vi "Eurotherm_read_TH.vi"(0 "Modbus Master in":refnum<class "Modbus Master.lvclass">, 5 "error in (no error)":errorcluster) -> (12 "HR_rd":dbl min=-28.0 max=70.0 step=0.1, 14 "Modbus Master out":refnum<class "Modbus Master.lvclass">, 18 "Tª_rd":dbl min=-28.0 max=70.0 step=0.1, 19 "error out":errorcluster)   [LabVIEW 2021, in "CC_Library.lvlib"]
uses:
  CC_Library.lvlib
  <vilib>/Modbus/master/Modbus Master.lvclass
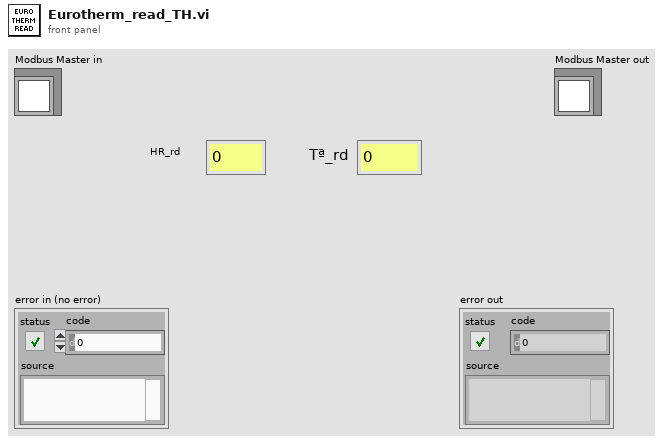
[diagram p1: front panel]
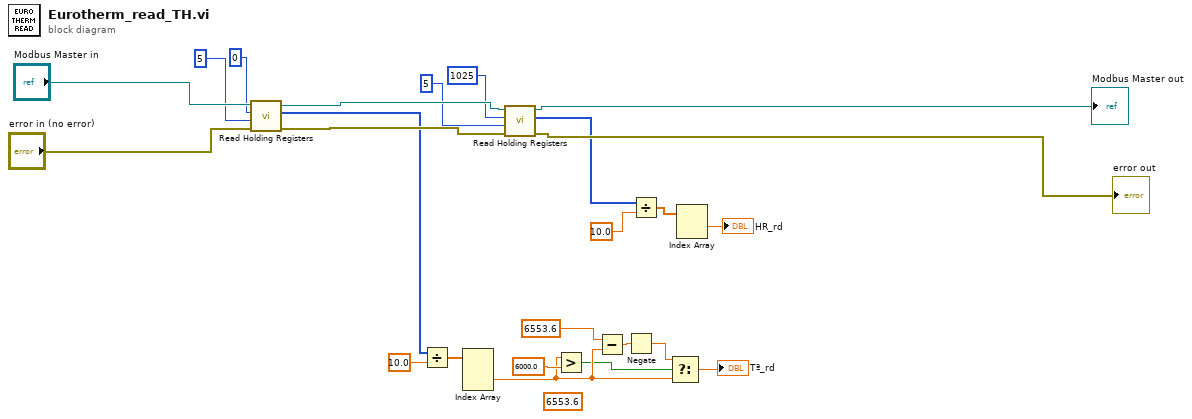
[diagram p0: block diagram]
diagram:
  (unwired) 6553.6 ("x")
  n1 = call-dynamic "Read Holding Registers.vi"("error in (no error)"="error in (no error)", "number of holding registers"=u16 5, "starting address"=u16 0 ("address"), "Modbus master in"="Modbus Master in") -> ("error out"=w21:errorcluster, "register values"=w20:u16[], "Modbus master out"=w22:refnum<class "Modbus Master.lvclass">)  [unwired: 5 in]
  n2 = Divide(x=w20, y=10.0) -> (x/y=w8:dbl[])
  n3 = Index Array(array=w8) -> (element #2=w11:dbl)  [unwired: 3 in, 2 out]
  n4 = call-dynamic "Read Holding Registers.vi"("error in (no error)"=w21, "number of holding registers"=u16 5 ("number of holding registers 2"), "starting address"=u16 1025 ("address"), "Modbus master in"=w22) -> ("error out"=→"error out":errorcluster, "register values"=w3:u16[], "Modbus master out"=→"Modbus Master out":refnum<class "Modbus Master.lvclass">)  [unwired: 5 in]
  n5 = Greater?(x=w11, y=6000.0) -> (0:w9:bool)
  n6 = Subtract(x=6553.6, y=w11) -> (x-y=w13:dbl)
  n7 = Negate(x=w13) -> (-x=w10:dbl)
  n8 = Divide(x=w3, y=10.0) -> (x/y=w5:dbl[])
  n9 = Select(t=w10, s=w9, f=w11) -> (s? t:f=→"Tª_rd":dbl)
  n10 = Index Array(array=w5) -> (element #1=→"HR_rd":dbl)  [unwired: 2 in, 1 out]
